vi "StateObserverFeedback.vi"() -> ()   [LabVIEW 2016]
uses:
  <vilib>/Analysis/Matrix/Datatypes/RealMatrix.ctl
  <vilib>/Simulation/Scripting/Companion Diagram/SimConfigNode/SimParams.ctl
  <vilib>/Simulation/Scripting/Companion Diagram/SimConfigNode/_simSolvers.ctl
  <vilib>/Simulation/Implementation/Shared/SIMSCR Execution Mode.ctl
  <vilib>/Platform/TimedLoop/XDataNode/timing_clust.ctl
  <vilib>/Platform/TimedLoop/XDataNode/nitl_modes.ctl
  <vilib>/Platform/TimedLoop/XDataNode/wakeup.ctl
  <vilib>/Simulation/Param Hierarchy/Typedefs/SIMPH Param Control Actions.ctl
  <vilib>/Simulation/Implementation/Shared/NILVSim_ParamChanged.vi
  <vilib>/Simulation/Implementation/Shared/NILVSim_FinishedLate.vi
  <vilib>/Simulation/Implementation/Shared/NILVSIM_BeginStep.vi
  <vilib>/Simulation/Utility/Implementation/SIM Halt.vi
  <vilib>/Simulation/Utility/Implementation/NILVSim Collector.llb/SIM Collector (scalar).vi
  <vilib>/Simulation/DiscreteLinear/Implementation/NILVSim Discrete Delay.llb/NILVSim Discrete Delay Buffered Distributor (vector).vi
  <vilib>/Analysis/baseanly.llb/A x B.vi
  <vilib>/Analysis/baseanly.llb/A x Vector.vi
  <vilib>/Simulation/Implementation/Shared/SIM Is Init or Final Stage.vi
  <vilib>/Simulation/DataSources/Implementation/NILVSim Sine Wave.llb/SIM Sine Wave (scalar).vi
  <vilib>/Simulation/DataSources/Implementation/NILVSim Ramp.llb/SIM Ramp (scalar).vi
  <vilib>/Simulation/DataSources/Implementation/NILVSim Step.llb/SIM Step (scalar).vi
  <vilib>/Simulation/DataSources/Implementation/NILVSim Chirp Signal.llb/SIM Chirp Signal (scalar).vi
  <vilib>/Simulation/Nonlinear/Implementation/NILVSim Saturation.llb/SIM Saturation (scalar).vi
  <vilib>/Simulation/DiscreteLinear/Implementation/NILVSim Discrete Delay.llb/NILVSim Discrete Delay Buffered Collector (vector).vi
  <vilib>/Simulation/Implementation/Shared/NILVSim_Manager.vi
  <vilib>/Utility/error.llb/Clear Errors.vi
  <vilib>/Simulation/Implementation/Shared/NILVSim_FinalizeModel.vi
  <vilib>/Simulation/Utility/Implementation/NILVSim Collector.llb/NILVSim Collector core (scalar).vi
  <vilib>/Simulation/Implementation/Shared/SIM Unbundle Sim Info.vi
  <vilib>/Simulation/Implementation/Shared/SIMSH Read Queue.vi
  <vilib>/Simulation/Implementation/Shared/NILVSim_Initialize.vi
  SubVI/StateObserver.vi
  SubVI/CommandDuty.vi
  <vilib>/Simulation/Utility/Implementation/NILVSim Get Time and IsAcceptedStep.vi
  <vilib>/Simulation/Implementation/Shared/NILVSim_GetModelError.vi
  <vilib>/Simulation/Implementation/Shared/SIM Bundle Sim Info.vi
  <vilib>/Simulation/Scripting/Companion Diagram/SimConfigNode/SimDog.xnode
  <vilib>/Platform/TimedLoop/XDataNode/XDataNode.xnode
  <vilib>/Simulation/Implementation/XNodeFramework/SimXNode/SimX.xnode
  <vilib>/Analysis/NI_AALBase.lvlib
  <vilib>/Simulation/DiscreteLinear/Implementation/NILVSim Discrete Delay.llb/SIM Discrete Delay Buffered (vector).vi
  <vilib>/Platform/TimedLoop/XDataNode/XDNodeRunTimeDep.lvlib
  <vilib>/Simulation/Implementation/Shared/NI_SIM_Implementation.lvlib
  <vilib>/Analysis/Matrix/NI_Matrix.lvlib
panel:
  in  "Tab Control":enum32{"Motor Control", "Debug"}(tab)
  in  "Amplitude":dbl=0.2
  in  "Input Type":string(combo)="Chirp"
  in  "Run Control":bool
  out "Reference r and Output y":cluster{"Constant":dbl, dbl}(graph)
  out "Control input u":dbl(graph)
  in  "Final Time (s)":dbl=10.0
  in  "Saturation Amp":dbl=1.0
  in  "K":T1=[[4.67, 70.57]]
  in  "FF gain":dbl=0.00361845
  in  "L":dbl[](array[numeric])=[2.925, 0.279]
  in  "Pc":T1=[[0.0, 2.15]]
  in  "Pb":dbl[](array[numeric])=[0.1281, 0.0001]
  in  "Pa":T1=[[1.0012, 0.0117], [0.016, 1.0001]]
  in  "Ts":dbl
  out "Counter Value":i32
  out "error out":errorcluster
  out "Error":errorcluster
  # "Control Settings"
  # "Data Logging"
  # "Hint: You don't need to do anything in this page"
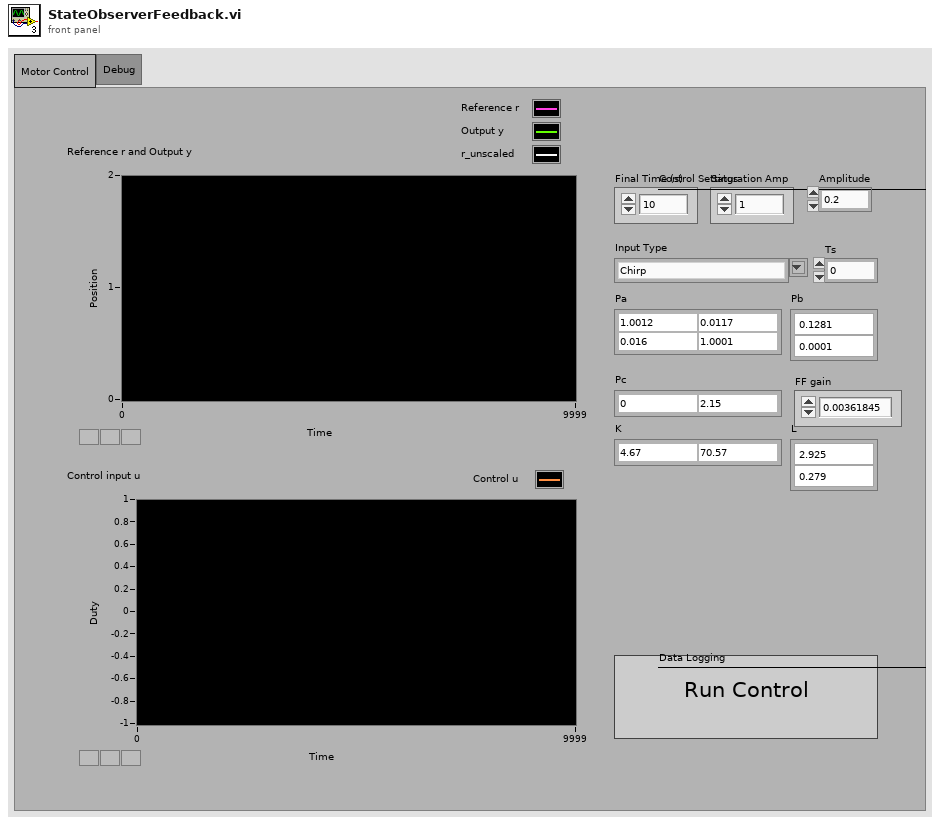
[diagram p1: front panel]
types:
  T1 = typedef "NI_Matrix.lvlib/RealMatrix.ctl" = dbl[][]
  T2 = typedef "SIMSCR Execution Mode.ctl" = enum16{"Simulate to Completion", "Single Time-Step Simulation (Fixed Step Only)"}
  T3 = typedef "XDNodeRunTimeDep.lvlib/timing_clust.ctl" = cluster{"Expected End [f-1]":u64, "Actual End [f-1]":u64, "Finished Late? [f-1]":bool, "Expected End [i-1]":u64, "Actual End [i-1]":u64, "Finished Late? [i-1]":bool, "Expected Start [i]":u64, "Actual Start [i]":u64, "Expected Start [f]":u64, "Actual Start [f]":u64, "Source Name":string, "Structure Name":string, "Period":i64, "Deadline":i64, "Offset":i64, "Start":i64, "Priority":i32, "Timeout":i32, "Mode":T4, "Wakeup Reason":T5, "Error":errorcluster, "Source Type":string, "Secondary Source Type":string, "Global End Time":u64, "Global Start Time":u64, "Frame Duration":u64, "Iteration Duration":u64, "Assigned CPU":i32, "I/O Scan Engine Mode":u32}
  T4 = typedef "XDNodeRunTimeDep.lvlib/nitl_modes.ctl" = enum32{"No Change", "Process missed periods, maintain original phase", "Discard missed periods, maintain original phase", "Process missed periods, ignore original phase", "Discard missed periods, ignore original phase"}
  T5 = typedef "XDNodeRunTimeDep.lvlib/wakeup.ctl" = enum32{"Normal", "Aborted", "Asynchronous wakeup", "Timing source error", "Timed loop error", "Timeout"}
  T6 = typedef "SIMPH Param Control Actions.ctl" = enum16{"get params", "set params"}
  T7 = typedef "SimParams.ctl" = cluster{"Initial Time (s)":dbl, "Final Time (s)":dbl, "Step Size (s)":dbl, "ODE Solver":T8, "Minimum Step Size (s)":dbl, "Maximum Step Size (s)":dbl, "Relative Tolerance":dbl, "Absolute Tolerance":dbl, "Software Timing":bool, "Initial Step Size (s)":dbl, "Automatic Fixed Step Size?":bool, "Automatic Discrete Step Size?":bool, "Discrete Step Size (s)":dbl, "Calculate using Time Step":bool, "Solver Wired?":bool, "Prev.Frm.Expected End":u64, "Prev.Frm.Actual End":u64, "Prev.Frm.Finished Late?":bool, "Prev.Iter.Expected End":u64, "Prev.Iter.Actual End":u64, "Prev.Iter.Finished Late?":bool, "Expected Iteration Start":u64, "Actual Iteration Start":u64, "Expected Frame Start":u64, "Actual Frame Start":u64, "Source Name":string, "Name":string, "Period":i64, "Deadline":i64, "Offset":i64, "Start":i64, "Priority":i32, "Timeout":i32, "Processor":i32, "Mode":enum32{"No Change", "Process missed periods, maintain original phase", "Discard missed periods, maintain original phase", "Process missed periods, ignore original phase", "Discard missed periods, ignore original phase"}, "Wakeup reason":enum32{"Normal", "Aborted", "Asynchronous wakeup", "Timing source error", "Timed loop error", "Timeout"}, "Error":errorcluster, "Source Type":string, "Secondary Source Type":string, "Global End Time":u64, "Global Start Time":u64, "Full Solver Reset":bool, "Execution Mode":T2, "Nan/Inf Check":bool, "Custom Solver Library":string, "Solver Is Variable":bool, "custom solver name":string, "Signal Collection Decimation":u32}
  T8 = typedef "_simSolvers.ctl" = enum16{"Runge-Kutta 1 (Euler)", "Runge-Kutta 2", "Runge-Kutta 3", "Runge-Kutta 4", "Runge-Kutta 23 (variable)", "Runge-Kutta 45 (variable)", "BDF (variable)", "Adams-Moulton (variable)", "Rosenbrock (variable)", "Discrete States Only", "SDIRK 4 (variable)", "Radau 5 (variable)", "Radau 9 (variable)", "Radau 13 (variable)", "Radau [Variable Order] (variable)", "Gear's Method (variable)", "Linearizer", "State Query", "Trim Eval", "Custom Solver"}
  T9 = typedef "PWM.lvlib/PWM Reference.ctl" = cluster{"myRIO Reference":T10, "PWM Channels Enum":T14, "PWM Configuration":T15}
  T10 = typedef "myRIO Generic Hardware Reference.ctl" = cluster{"myRIO Model":T11, "myRIO Hardware Reference":T12}
  T11 = typedef "Hardware Version Enum.ctl" = enum16{"Unknown", "myRIO-1900", "myRIO-1950", "roboRIO", "NI ELVIS RIO CM"}
  T12 = typedef "myRIO v1.0 Reference.ctl" = cluster{"Generic FPGA Reference":T13, "Allow multiple opens":bool}
  T13 = typedef "Generic FPGA Reference.ctl" = refnum<k20>
  T14 = typedef "PWM Channels Enum.ctl" = enum16{"Not Connected", "C/PWM0", "C/PWM1", "A/PWM0", "A/PWM1", "A/PWM2", "B/PWM0", "B/PWM1", "B/PWM2", "PWM/PWM0", "PWM/PWM1", "PWM/PWM2", "PWM/PWM3", "PWM/PWM4", "PWM/PWM5", "PWM/PWM6", "PWM/PWM7", "PWM/PWM8", "PWM/PWM9"}
  T15 = typedef "PWM.lvlib/PWM Configuration.ctl" = cluster{"Frequency":dbl, "Duty Cycle":dbl}
  T16 = typedef "Encoder.lvlib/Encoder Reference.ctl" = cluster{"myRIO Reference":T10, "Encoder Channels Enum":T17}
  T17 = typedef "Encoder Channels Enum.ctl" = enum16{"Not Connected", "C/ENC0", "C/ENC1", "A/ENC", "B/ENC", "DIO/ENC0", "DIO/ENC1", "DIO/ENC2", "DIO/ENC3", "DIO/ENC4"}
  T18 = typedef "DIO.lvlib/DIO Reference.ctl" = cluster{"myRIO Reference":T10, "DIO Channels List":T19}
  T19 = typedef "DIO Channels List.ctl" = T20[]
  T20 = typedef "DIO Channels Enum.ctl" = enum16{"Not Connected", "C/DIO0", "C/DIO1", "C/DIO2", "C/DIO3", "C/DIO4", "C/DIO5", "C/DIO6", "C/DIO7", "A/DIO0", "A/DIO1", "A/DIO2", "A/DIO3", "A/DIO4", "A/DIO5", "A/DIO6", "A/DIO7", "A/DIO8", "A/DIO9", "A/DIO10", "A/DIO11", "A/DIO12", "A/DIO13", "A/DIO14", "A/DIO15", "B/DIO0", "B/DIO1", "B/DIO2", "B/DIO3", "B/DIO4", "B/DIO5", "B/DIO6", "B/DIO7", "B/DIO8", "B/DIO9", "B/DIO10", "B/DIO11", "B/DIO12", "B/DIO13", "B/DIO14", "B/DIO15", "LED0", "LED1", "LED2", "LED3", "Button0", "DIO/DIO0", "DIO/DIO1", "DIO/DIO2", "DIO/DIO3", "DIO/DIO4", "DIO/DIO5", "DIO/DIO6", "DIO/DIO7", "DIO/DIO8", "DIO/DIO9", "SPI/CS0", "SPI/CS1", "SPI/CS2", "SPI/CS3", "LED RADIO (Green)", "LED RADIO (Red)", "LED COMM (Green)", "LED COMM (Red)", "LED MODE (Green)", "LED MODE (Red)"}
  T21 = cluster{"PWM0":T9, "PWM1":T9, "Encoder":T16, "En":T18}
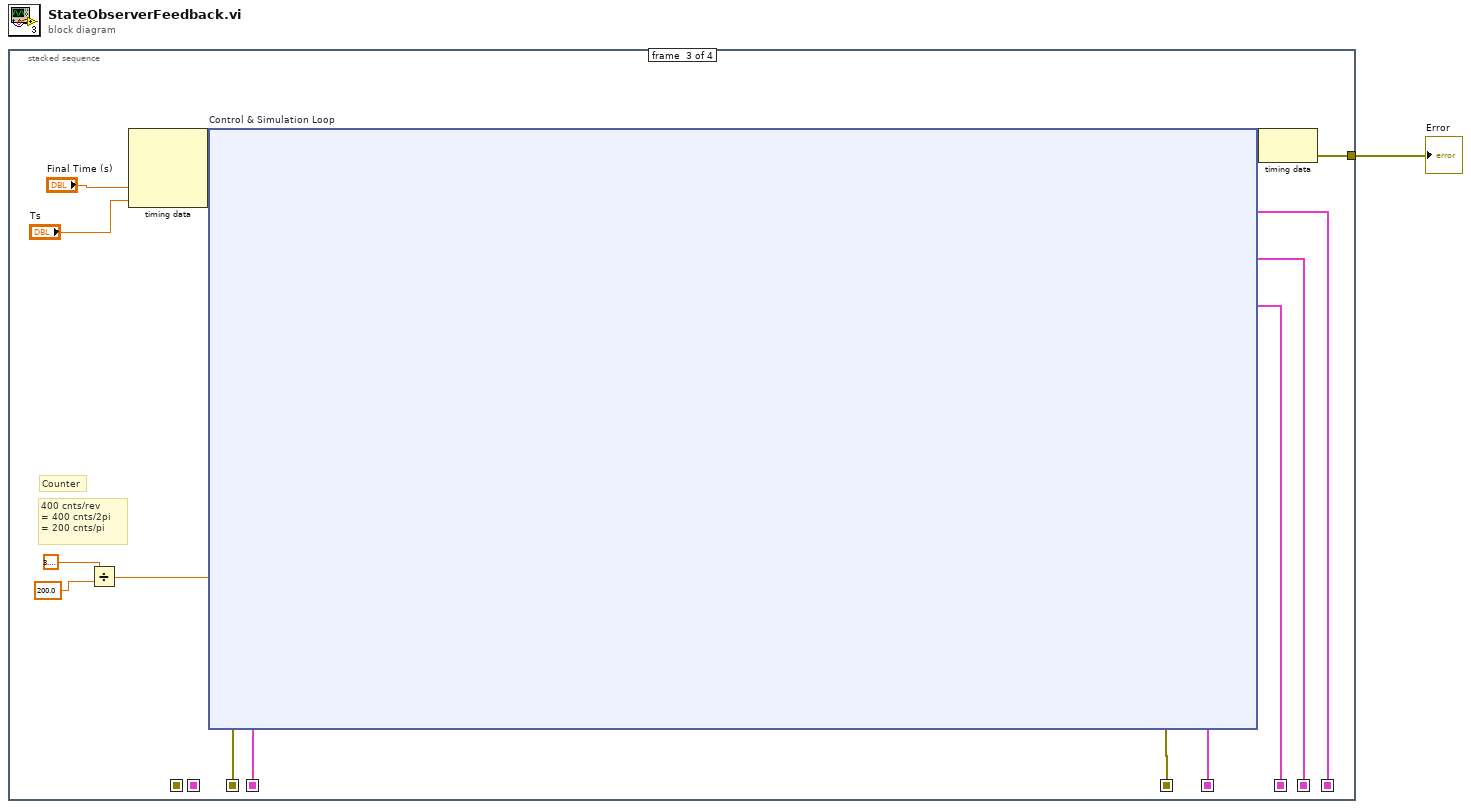
[diagram p0: block diagram]
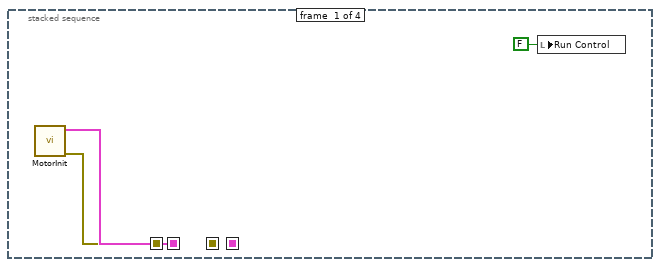
[diagram p2: hidden frame]
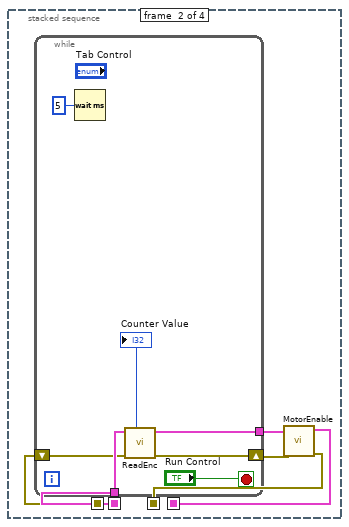
[diagram p3: hidden frame]
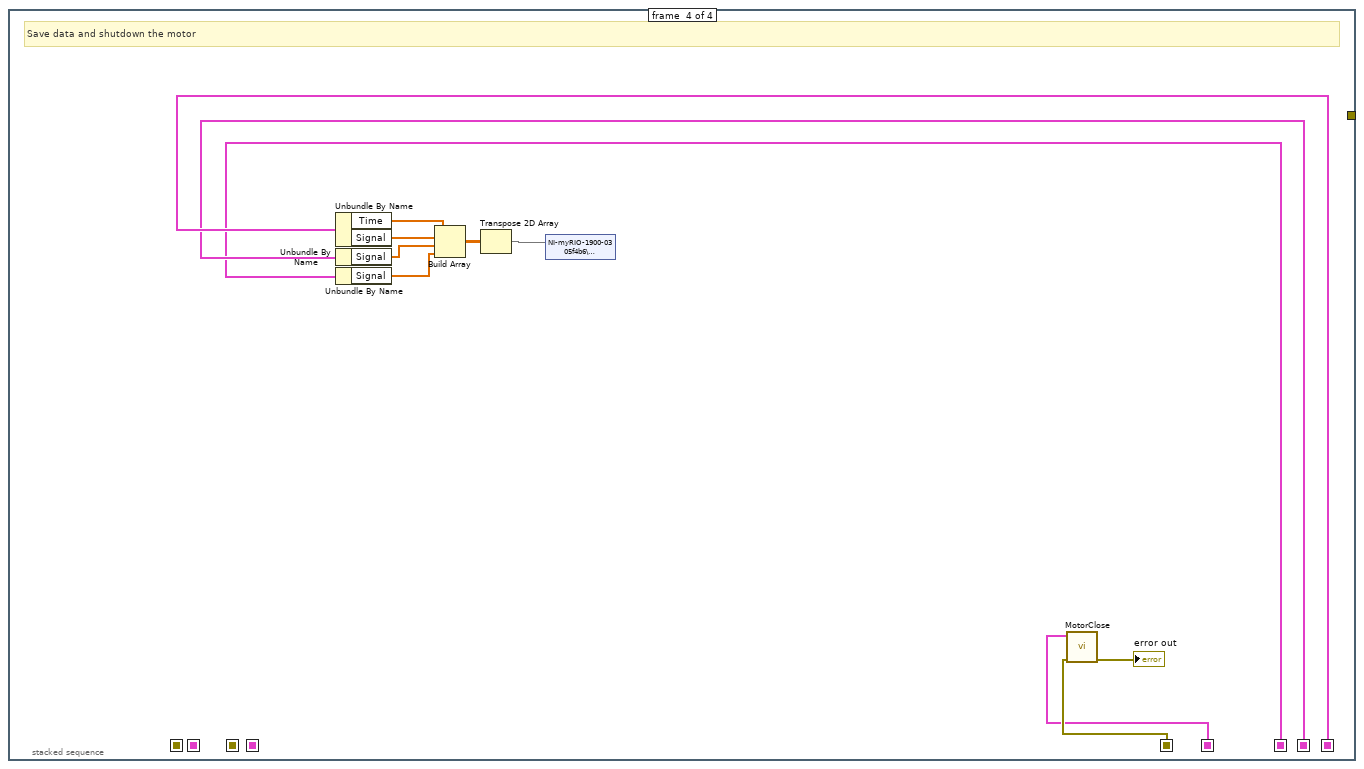
[diagram p4: hidden frame]
diagram:
  n1 = stacked-sequence {
    seq-local: [w3 _ _ _] -> [_ w10 _ _]
    seq-local: [w2 _ _ _] -> [_ w9 _ _]
    seq-local: [_ w6 _ _] -> [_ _ w27 _]
    seq-local: [_ w5 _ _] -> [_ _ w28 _]
    seq-local: [_ _ w25 _] -> [_ _ _ w715]
    seq-local: [_ _ w24 _] -> [_ _ _ w714]
    seq-local: [_ _ w21 _] -> [_ _ _ w709]
    seq-local: [_ _ w22 _] -> [_ _ _ w710]
    seq-local: [_ _ w23 _] -> [_ _ _ w713]
    tunnel: [_ _ w20 _] -> w1
    frame #0 {
      n2 = call "MotorInit.vi"() -> ("error out"=w2:errorcluster, "Cluster"=w3:T21)  [unwired: 10 in]
      n3 = local write "Run Control"(FALSE ("Run Control")) -> ()
    }
    frame #1 {
      n4 = while {
        tunnel: w10 -> [w16]
        shift-right: [w14] -> w7
        shift-left: w9 -> [w15]
        tunnel: [w13] -> w8
        stop <- "Run Control" stop-if-true
        n5 = Wait (ms)(milliseconds to wait=u32 5) -> ()  [unwired: 1 out]
        n6 = call "ReadEnc.vi"("error in"=w15, "Cluster In"=w16) -> ("error out"=w14:errorcluster, "Enc value [count]"=→"Counter Value":i32, "Cluster Out"=w13:T21)  [unwired: 7 in]
      }
      n7 = call "MotorEnable.vi"("error in"=w7, "Cluster In"=w8) -> ("error out"=w6:errorcluster, "Cluster Out"=w5:T21)  [unwired: 8 in]
    }
    frame #2 {
      # "Counter"
      # "400 cnts/rev\n= 400 cnts/2pi \n= 200 cnts/pi"
      n8 = Divide(x=3.141592653589793, y=200.0) -> (x/y=w26:dbl)
      n9 = node-c288("Final Time (s)", "Ts") -> (w30:variant)  [unwired: 2 in]
      n10 = node-c254 "Control & Simulation Loop"(w30, w28, w27, w26) -> (w29:variant, w25:errorcluster, w24:T21, w23:cluster{"Time":dbl[], "Signal":dbl[]}, w22:cluster{"Time":dbl[], "Signal":dbl[]}, w21:cluster{"Time":dbl[], "Signal":dbl[]})
      n11 = node-c288(w29) -> (w20:errorcluster)
    }
    frame #3 {
      # "Save data and shutdown the motor"
      n12 = Unbundle By Name(w713) -> ("Time"=w712:dbl[], "Signal"=w711:dbl[])
      n13 = Unbundle By Name(w710) -> ("Signal"=w708:dbl[])
      n14 = Unbundle By Name(w709) -> ("Signal"=w707:dbl[])
      n15 = Build Array(w712, w711, w708, w707) -> (w717:dbl[][])
      n16 = Transpose 2D Array(2D array=w717) -> (transposed array=w716:dbl[][])
      n17 = shared-variable "NI-myRIO-1900-0305f4b6\\MyVariables.lvlib\\Data"(w716) -> ()  [unwired: 1 in, 1 out]
      n18 = call "MotorClose.vi"("error in (no error)"=w715, "Cluster"=w714) -> ("error out"=→"error out":errorcluster)  [unwired: 9 in]
    }
  }
  "Error" <- w1
